vi "constructor.vi"(0 "Surface in":refnum<class "Surface.lvclass">, 1 "Color Matrix":sgl[][](array[numeric]), 5 "X vector":sgl[](array[numeric]), 7 "Y vector":sgl[](array[numeric]), 9 "Z Matrix":sgl[][](array[numeric]), 11 "error in (no error)":errorcluster, 12 "Plot ID":i32) -> (4 "Surface out":refnum<class "Surface.lvclass">, 15 "error out":errorcluster)   [LabVIEW 2020, in "Surface.lvclass"]
uses:
  <vilib>/Native 3D Graph/classes/Surface/Surface.lvclass
  <vilib>/Native 3D Graph/classes/Surface/Surface.lvclass/Surface.ctl
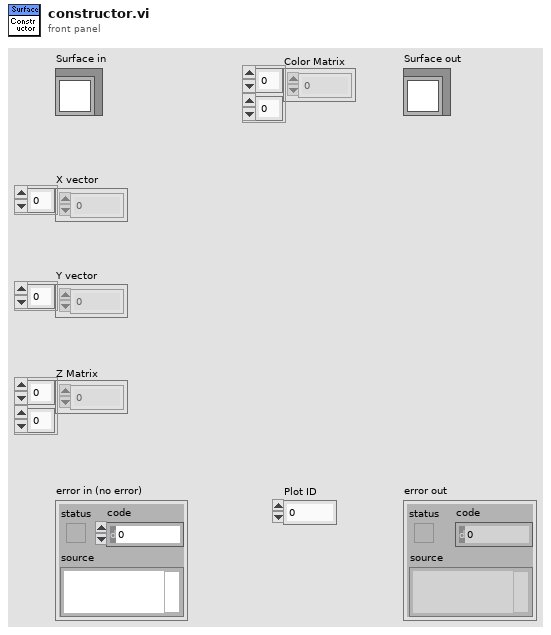
[diagram p1: front panel]
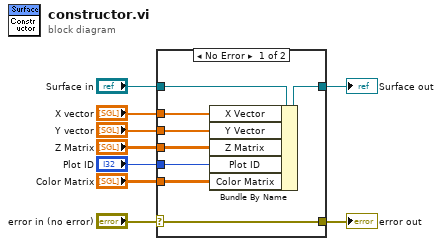
[diagram p0: block diagram]
diagram:
  n1 = case shown="No Error" "error in (no error)" {
    selector: "error in (no error)" -> [w17 w19]
    tunnel: [w17 w19] -> w8
    tunnel: [w15 w18] -> w7
    tunnel: "Surface in" -> [w16 w18]
    tunnel: "Color Matrix" -> [w14 _]
    tunnel: "Plot ID" -> [w13 _]
    tunnel: "Y vector" -> [w12 _]
    tunnel: "X vector" -> [w11 _]
    tunnel: "Z Matrix" -> [w10 _]
    frame No Error {
      n2 = Bundle By Name(cluster=w16, "X Vector"=w11, "Y Vector"=w12, "Z Matrix"=w10, "Plot ID"=w13, "Color Matrix"=w14) -> (w15:refnum<class "Surface.lvclass">)
    }
    frame Error {
    }
  }
  "error out" <- w8
  "Surface out" <- w7
